vi "calculator.vi"() -> ()   [LabVIEW 2012]
uses:
  <vilib>/gmath/NI_Gmath.lvlib
panel:
  in  "CE":bool
  in  ")":bool
  in  "(":bool
  out "SAVE 2":dbl
  out "SAVE 1":dbl
  in  "SAVE2":bool
  in  "SAVE1":bool
  in  "Backspace":bool
  in  "Sqrt":bool
  in  "1/x":bool
  in  "+/-":bool
  in  ".":bool
  out "String":string
  in  "stop":bool
  out "?":timestamp
  in  "=":bool
  out "Answer":dbl caption="left"
  in  "/":bool
  in  "x":bool
  in  "-":bool
  in  "+":bool
  in  "C":bool
  in  "OK Button 10":bool
  in  "OK Button 9":bool
  in  "OK Button 8":bool
  in  "OK Button 7":bool
  in  "OK Button 6":bool
  in  "OK Button 5":bool
  in  "OK Button 4":bool
  in  "OK Button 3":bool
  in  "OK Button 2":bool
  in  "OK Button":bool
  out "1/10cnt":dbl
  out "counter":dbl
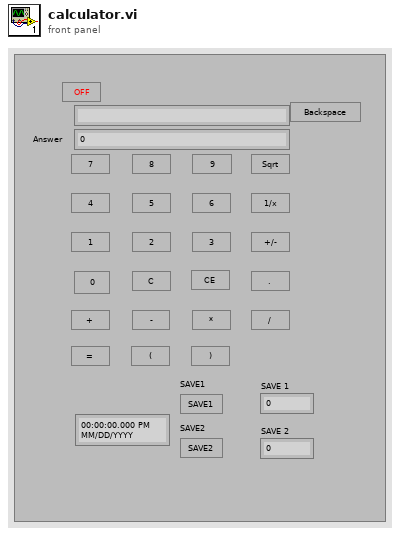
[diagram p1: front panel]
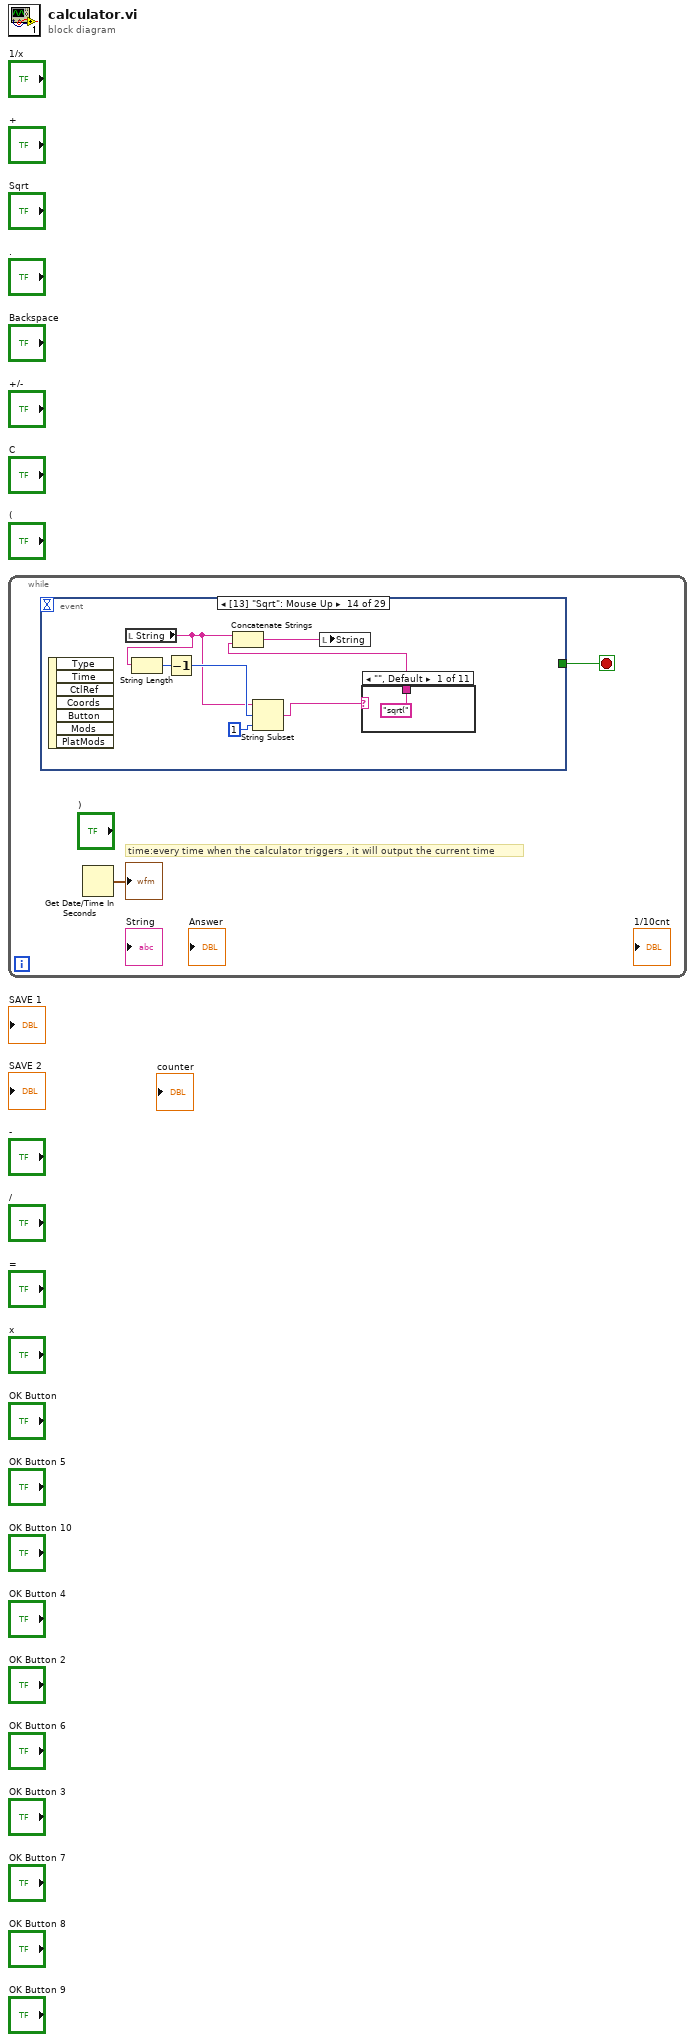
[diagram p0: block diagram]
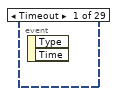
[diagram p2: hidden frame]
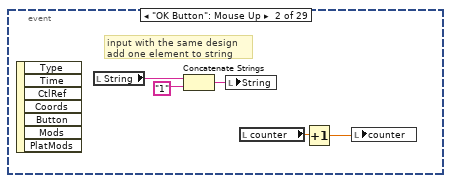
[diagram p3: hidden frame]
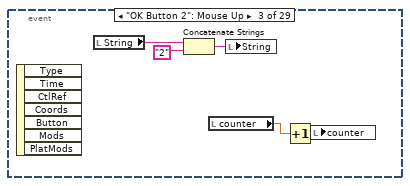
[diagram p4: hidden frame]
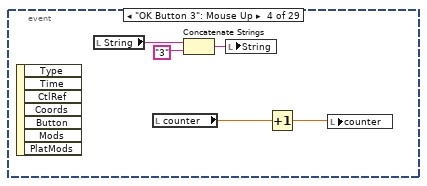
[diagram p5: hidden frame]
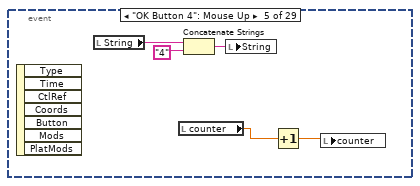
[diagram p6: hidden frame]
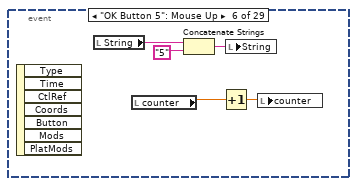
[diagram p7: hidden frame]
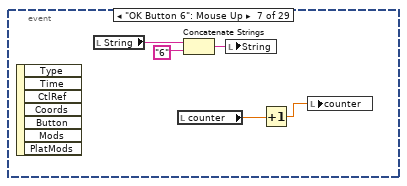
[diagram p8: hidden frame]
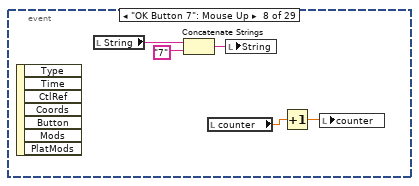
[diagram p9: hidden frame]
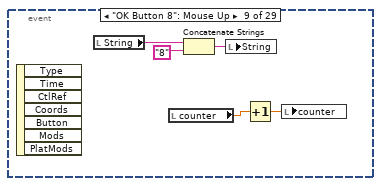
[diagram p10: hidden frame]
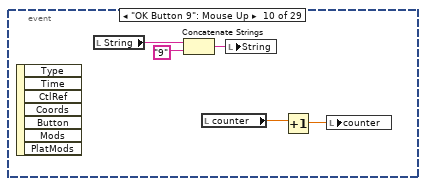
[diagram p11: hidden frame]
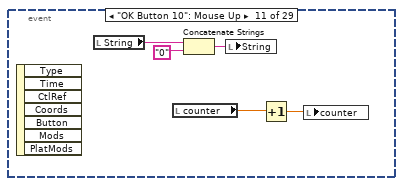
[diagram p12: hidden frame]
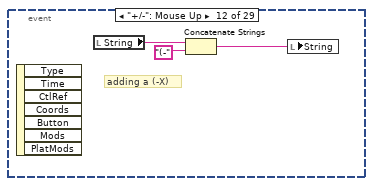
[diagram p13: hidden frame]
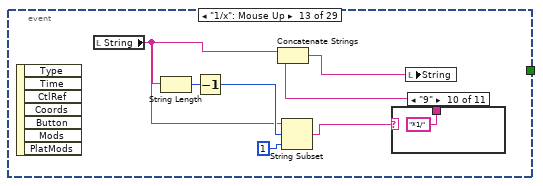
[diagram p14: hidden frame]
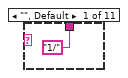
[diagram p15: hidden frame]
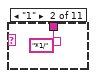
[diagram p16: hidden frame]
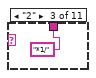
[diagram p17: hidden frame]
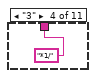
[diagram p18: hidden frame]
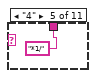
[diagram p19: hidden frame]
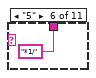
[diagram p20: hidden frame]
diagram:
  n1 = while {
    stop <- w2 stop-if-true
    # "time:every time when the calculator triggers , it will output the current time"
    n2 = event shown="[13] \"Sqrt\": Mouse Up" {
      selector: _ -> [_ _ _ _ _ _ _ _ _ _ _ _ _ _ _ _ _ _ _ _ _ _ _ _ _ _ _ _ _]
      dyn-events: _ -> [_ _ _ _ _ _ _ _ _ _ _ _ _ _ _ _ _ _ _ _ _ _ _ _ _ _ _ _ _]
      timeout: _ -> [_ _ _ _ _ _ _ _ _ _ _ _ _ _ _ _ _ _ _ _ _ _ _ _ _ _ _ _ _]
      tunnel: [_ _ _ _ _ _ _ _ _ _ _ _ _ _ _ _ _ _ _ _ _ _ _ _ _ _ _ w134 _] -> w2
      event Timeout {
        n3 = event-data() -> ()  [unwired: 1 in, 2 out]
      }
      event "OK Button": Mouse Up {
        # "input with the same design\nadd one element to string"
        n4 = event-data() -> ()  [unwired: 1 in, 7 out]
        n5 = local read "String"() -> (w5:string)
        n6 = Concatenate Strings(w5, "1") -> (w6:string)
        n7 = local write "String"(w6) -> ()
        n8 = local read "counter"() -> (w3:dbl)
        n9 = Increment(x=w3) -> (x+1=w4:dbl)
        n10 = local write "counter"(w4) -> ()
      }
      event "OK Button 2": Mouse Up {
        n11 = event-data() -> ()  [unwired: 1 in, 7 out]
        n12 = local read "String"() -> (w10:string)
        n13 = Concatenate Strings(w10, "2") -> (w11:string)
        n14 = local read "counter"() -> (w9:dbl)
        n15 = local write "String"(w11) -> ()
        n16 = Increment(x=w9) -> (x+1=w8:dbl)
        n17 = local write "counter"(w8) -> ()
      }
      event "OK Button 3": Mouse Up {
        n18 = event-data() -> ()  [unwired: 1 in, 7 out]
        n19 = local read "String"() -> (w16:string)
        n20 = local read "counter"() -> (w14:dbl)
        n21 = Concatenate Strings(w16, "3") -> (w15:string)
        n22 = local write "String"(w15) -> ()
        n23 = Increment(x=w14) -> (x+1=w13:dbl)
        n24 = local write "counter"(w13) -> ()
      }
      event "OK Button 4": Mouse Up {
        n25 = event-data() -> ()  [unwired: 1 in, 7 out]
        n26 = local read "String"() -> (w20:string)
        n27 = local read "counter"() -> (w19:dbl)
        n28 = Concatenate Strings(w20, "4") -> (w21:string)
        n29 = local write "String"(w21) -> ()
        n30 = Increment(x=w19) -> (x+1=w18:dbl)
        n31 = local write "counter"(w18) -> ()
      }
      event "OK Button 5": Mouse Up {
        n32 = event-data() -> ()  [unwired: 1 in, 7 out]
        n33 = local read "String"() -> (w25:string)
        n34 = local read "counter"() -> (w23:dbl)
        n35 = Concatenate Strings(w25, "5") -> (w26:string)
        n36 = Increment(x=w23) -> (x+1=w24:dbl)
        n37 = local write "String"(w26) -> ()
        n38 = local write "counter"(w24) -> ()
      }
      event "OK Button 6": Mouse Up {
        n39 = event-data() -> ()  [unwired: 1 in, 7 out]
        n40 = local read "String"() -> (w30:string)
        n41 = local read "counter"() -> (w29:dbl)
        n42 = Concatenate Strings(w30, "6") -> (w31:string)
        n43 = local write "String"(w31) -> ()
        n44 = Increment(x=w29) -> (x+1=w28:dbl)
        n45 = local write "counter"(w28) -> ()
      }
      event "OK Button 7": Mouse Up {
        n46 = event-data() -> ()  [unwired: 1 in, 7 out]
        n47 = local read "String"() -> (w35:string)
        n48 = Concatenate Strings(w35, "7") -> (w36:string)
        n49 = local read "counter"() -> (w33:dbl)
        n50 = local write "String"(w36) -> ()
        n51 = Increment(x=w33) -> (x+1=w34:dbl)
        n52 = local write "counter"(w34) -> ()
      }
      event "OK Button 8": Mouse Up {
        n53 = event-data() -> ()  [unwired: 1 in, 7 out]
        n54 = local read "String"() -> (w40:string)
        n55 = local read "counter"() -> (w38:dbl)
        n56 = Concatenate Strings(w40, "8") -> (w41:string)
        n57 = local write "String"(w41) -> ()
        n58 = Increment(x=w38) -> (x+1=w39:dbl)
        n59 = local write "counter"(w39) -> ()
      }
      event "OK Button 9": Mouse Up {
        n60 = event-data() -> ()  [unwired: 1 in, 7 out]
        n61 = local read "String"() -> (w45:string)
        n62 = Concatenate Strings(w45, "9") -> (w46:string)
        n63 = local read "counter"() -> (w43:dbl)
        n64 = local write "String"(w46) -> ()
        n65 = Increment(x=w43) -> (x+1=w44:dbl)
        n66 = local write "counter"(w44) -> ()
      }
      event "OK Button 10": Mouse Up {
        n67 = event-data() -> ()  [unwired: 1 in, 7 out]
        n68 = local read "String"() -> (w50:string)
        n69 = local read "counter"() -> (w48:dbl)
        n70 = Concatenate Strings(w50, "0") -> (w51:string)
        n71 = local write "String"(w51) -> ()
        n72 = Increment(x=w48) -> (x+1=w49:dbl)
        n73 = local write "counter"(w49) -> ()
      }
      event "+/-": Mouse Up {
        # "adding a (-X)"
        n74 = event-data() -> ()  [unwired: 1 in, 7 out]
        n75 = local read "String"() -> (w53:string)
        n76 = Concatenate Strings(w53, "(-") -> (w54:string)
        n77 = local write "String"(w54) -> ()
      }
      event "1/x": Mouse Up {
        n78 = event-data() -> ()  [unwired: 1 in, 7 out]
        n79 = local read "String"() -> (w58:string)
        n80 = String Length(string=w58) -> (length=w61:i32)
        n81 = Decrement(x=w61) -> (x-1=w60:i32)
        n82 = String Subset(string=w58, offset (0)=w60, length (rest)=1) -> (substring=w57:string)
        n83 = case shown="\"9\"" w57 {
          tunnel: ["1/" "*1/" "*1/" "*1/" "*1/" "*1/" "*1/" "*1/" "*1/" "*1/" "*1/"] -> w56
          frame "", Default {
          }
          frame "1" {
          }
          frame "2" {
          }
          frame "3" {
          }
          frame "4" {
          }
          frame "5" {
          }
          frame "6" {
          }
          frame "7" {
          }
          frame "8" {
          }
          frame "9" {
          }
          frame "0" {
          }
        }
        n84 = Concatenate Strings(w58, w56) -> (w62:string)
        n85 = local write "String"(w62) -> ()
      }
      event "Sqrt": Mouse Up {
        n86 = event-data() -> ()  [unwired: 1 in, 7 out]
        n87 = local read "String"() -> (w74:string)
        n88 = String Length(string=w74) -> (length=w77:i32)
        n89 = Decrement(x=w77) -> (x-1=w78:i32)
        n90 = String Subset(string=w74, offset (0)=w78, length (rest)=1) -> (substring=w76:string)
        n91 = case shown="\"\", Default" w76 {
          tunnel: ["sqrt(" "*sqrt(" "*sqrt(" "*sqrt(" "*sqrt(" "*sqrt(" "*sqrt(" "*sqrt(" "*sqrt(" "*sqrt(" "*sqrt("] -> w75
          frame "", Default {
          }
          frame "1" {
          }
          frame "2" {
          }
          frame "3" {
          }
          frame "4" {
          }
          frame "5" {
          }
          frame "6" {
          }
          frame "7" {
          }
          frame "8" {
          }
          frame "9" {
          }
          frame "0" {
          }
        }
        n92 = Concatenate Strings(w74, w75) -> (w80:string)
        n93 = local write "String"(w80) -> ()
      }
      event "Backspace": Mouse Up {
        n94 = event-data() -> ()  [unwired: 1 in, 7 out]
        n95 = local read "String"() -> (w95:string)
        n96 = String Length(string=w95) -> (length=w93:i32)
        n97 = Decrement(x=w93) -> (x-1=w94:i32)
        n98 = String Subset(string=w95, offset (0)=0, length (rest)=w94) -> (substring=w96:string)
        n99 = local write "String"(w96) -> ()
      }
      event "C": Mouse Up {
        w97 = 0
        # "reset all"
        n100 = event-data() -> ()  [unwired: 1 in, 7 out]
        n101 = local write "Answer"(w97) -> ()
        n102 = local write "String"("") -> ()
        n103 = local write "counter"(w97) -> ()
      }
      event "CE": Mouse Up {
        n104 = event-data() -> ()  [unwired: 1 in, 7 out]
        n105 = local read "counter"() -> (w100:dbl)
        n106 = local read "String"() -> (w105:string)
        n107 = String Length(string=w105) -> (length=w104:i32)
        n108 = Subtract(x=w104, y=w100) -> (x-y=w103:dbl)
        n109 = String Subset(string=w105, length (rest)=w103) -> (substring=w102:string)  [unwired: 1 in]
        n110 = local read "counter"() -> (w101:dbl)
        n111 = local write "String"(w102) -> ()
        n112 = Subtract(x=w101, y=w100) -> (x-y=w99:dbl)
        n113 = local write "counter"(w99) -> ()
      }
      event "+": Mouse Up {
        # "all operators input to string"
        n114 = event-data() -> ()  [unwired: 1 in, 7 out]
        n115 = local read "String"() -> (w108:string)
        n116 = local write "counter"(0) -> ()
        n117 = Concatenate Strings(w108, "+") -> (w109:string)
        n118 = local write "String"(w109) -> ()
      }
      event "-": Mouse Up {
        n119 = event-data() -> ()  [unwired: 1 in, 7 out]
        n120 = local read "String"() -> (w112:string)
        n121 = Concatenate Strings(w112, "-") -> (w113:string)
        n122 = local write "String"(w113) -> ()
        n123 = local write "counter"(0) -> ()
      }
      event "x": Mouse Up {
        n124 = event-data() -> ()  [unwired: 1 in, 7 out]
        n125 = local read "String"() -> (w117:string)
        n126 = Concatenate Strings(w117, "*") -> (w116:string)
        n127 = local write "String"(w116) -> ()
        n128 = local write "counter"(0) -> ()
      }
      event "/": Mouse Up {
        n129 = event-data() -> ()  [unwired: 1 in, 7 out]
        n130 = local read "String"() -> (w121:string)
        n131 = Concatenate Strings(w121, "/") -> (w120:string)
        n132 = local write "String"(w120) -> ()
        n133 = local write "counter"(0) -> ()
      }
      event "=": Mouse Up {
        n134 = event-data() -> ()  [unwired: 1 in, 7 out]
        n135 = local read "String"() -> (w122:string)
        n136 = call <vilib>:"Eval Formula String.vi"("formula"=w122) -> ("y value"=w123:dbl)  [unwired: 1 in, 1 out]
        n137 = local write "Answer"(w123) -> ()
      }
      event "SAVE1": Mouse Up {
        n138 = event-data() -> ()  [unwired: 1 in, 7 out]
        n139 = local read "Answer"() -> (w124:dbl)
        n140 = local write "SAVE 1"(w124) -> ()
      }
      event "(": Mouse Up {
        n141 = event-data() -> ()  [unwired: 1 in, 7 out]
        n142 = local read "String"() -> (w128:string)
        n143 = Concatenate Strings(w128, "(") -> (w127:string)
        n144 = local write "String"(w127) -> ()
        n145 = local write "counter"(0) -> ()
      }
      event ")": Mouse Up {
        n146 = event-data() -> ()  [unwired: 1 in, 7 out]
        n147 = local read "String"() -> (w131:string)
        n148 = Concatenate Strings(w131, ")") -> (w132:string)
        n149 = local write "String"(w132) -> ()
        n150 = local write "counter"(0) -> ()
      }
      event "SAVE2": Mouse Up {
        n151 = event-data() -> ()  [unwired: 1 in, 7 out]
        n152 = local read "Answer"() -> (w133:dbl)
        n153 = local write "SAVE 2"(w133) -> ()
      }
      event Pane Size {
        n154 = event-data() -> ()  [unwired: 1 in, 5 out]
      }
      event "stop": Mouse Down {
        n155 = event-data() -> ()  [unwired: 1 in, 7 out]
        n156 = Not(x="stop") -> (.not. x?=w134:bool)
      }
      event ".": Mouse Up {
        n157 = event-data() -> ()  [unwired: 1 in, 7 out]
        n158 = local read "String"() -> (w136:string)
        n159 = Concatenate Strings(w136, ".") -> (w137:string)
        n160 = local write "String"(w137) -> ()
      }
    }
    n161 = Get Date/Time In Seconds() -> (seconds since 1Jan1904=→"?":timestamp)
  }
